vi "set_Fe.vi"(0 "Active":bool, 1 "Fe Flow 3":dbl, 2 "Fe Flow 2":dbl, 3 "Fe Flow 1":dbl, 5 "Bubbler":bool, 7 "H2 Dilute":bool, 9 "Run":bool, 11 "Remote":bool) -> ()   [LabVIEW 2011]
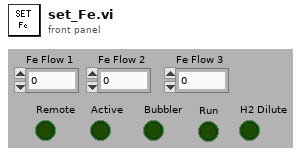
[diagram p1: front panel]
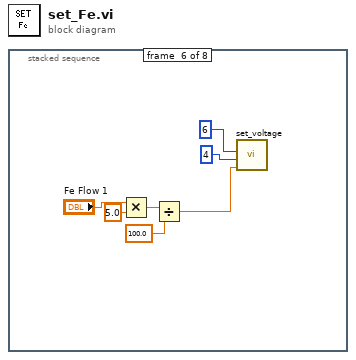
[diagram p0: block diagram]
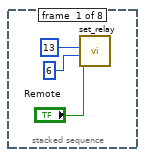
[diagram p2: hidden frame]
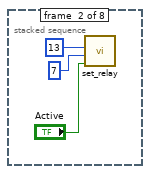
[diagram p3: hidden frame]
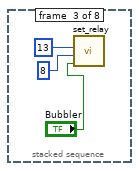
[diagram p4: hidden frame]
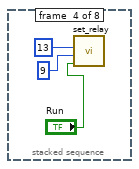
[diagram p5: hidden frame]
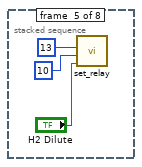
[diagram p6: hidden frame]
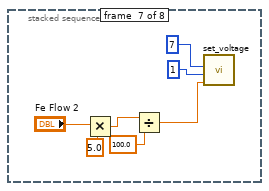
[diagram p7: hidden frame]
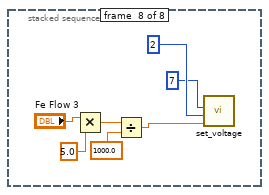
[diagram p8: hidden frame]
diagram:
  n1 = stacked-sequence {
    frame #0 {
      n2 = call "set_relay.vi"("Slot"=13, "Relay"=6, "Relay Status"="Remote") -> ()  [unwired: 2 in, 1 out]
    }
    frame #1 {
      n3 = call "set_relay.vi"("Slot"=13, "Relay"=7, "Relay Status"="Active") -> ()  [unwired: 1 in, 2 out]
    }
    frame #2 {
      n4 = call "set_relay.vi"("Slot"=13, "Relay"=8, "Relay Status"="Bubbler") -> ()  [unwired: 1 in, 2 out]
    }
    frame #3 {
      n5 = call "set_relay.vi"("Slot"=13, "Relay"=9, "Relay Status"="Run") -> ()  [unwired: 1 in, 2 out]
    }
    frame #4 {
      n6 = call "set_relay.vi"("Slot"=13, "Relay"=10, "Relay Status"="H2 Dilute") -> ()  [unwired: 1 in, 2 out]
    }
    frame #5 {
      n7 = Multiply(x="Fe Flow 1", y=5.0) -> (x*y=w19:dbl)
      n8 = Divide(x=w19, y=100.0) -> (x/y=w21:dbl)
      n9 = call "set_voltage.vi"("Voltage"=w21, "Channel Index"=4 ("Channel"), "Slot"=6) -> ()  [unwired: 1 in, 1 out]
    }
    frame #6 {
      n10 = Multiply(x="Fe Flow 2", y=5.0) -> (x*y=w26:dbl)
      n11 = Divide(x=w26, y=100.0) -> (x/y=w28:dbl)
      n12 = call "set_voltage.vi"("Voltage"=w28, "Channel Index"=1 ("Channel"), "Slot"=7) -> ()  [unwired: 1 in, 1 out]
    }
    frame #7 {
      n13 = Multiply(x="Fe Flow 3", y=5.0) -> (x*y=w33:dbl)
      n14 = Divide(x=w33, y=1000.0) -> (x/y=w35:dbl)
      n15 = call "set_voltage.vi"("Voltage"=w35, "Channel Index"=2 ("Channel"), "Slot"=7) -> ()  [unwired: 1 in, 1 out]
    }
  }
